vi "Settings Panel.vi"() -> ()   [LabVIEW 2012, in "Scan Driver.lvclass"]
doc: "Main method of the Scan Driver class. Construct a new Scan Driver instance from the given options, or load and deserialize one from an XML file, or modify the last run scan. Configure the instance. Run the scan, and repeat it if more than one scan is requested."
uses:
  Scan Driver.lvclass
  Scanner List.ctl
  Reader List.ctl
  Scan Setup Mode.ctl
  Scan Driver.lvclass/Scan Driver.ctl
  File IO/File IO.lvclass
  Global/File Locations.vi
panel:
  in  "Scanner 2":T1=enum."None"
  in  "Use LCD?":bool
  in  "Based on Last Scan":bool=TRUE
  in  "Path":path
  in  "Scanner":T1
  in  "Reader":T2
  in  "Scan Setup":T3
  out "Update UI":bool
  in  "Continue":bool
  out "error out":errorcluster
  in  "error in (no error)":errorcluster
  in  "exit":bool
  out "dispscan":string caption="Previous Settings"
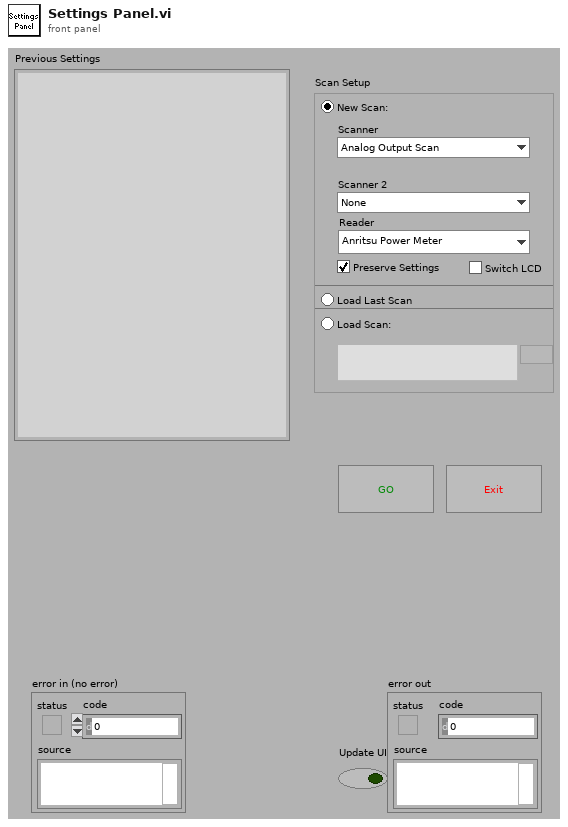
[diagram p1: front panel]
types:
  T1 = typedef "Scan Driver.lvclass/Scanner List.ctl" = enum16{"Analog Output Scan", "Continuous", "Dummy Scan", "Function Gen Scan", "Magnetic Field", "Magna Current Scan", "Magna Voltage Scan", "Microwave Freq Scan", "Pulse Gen Scan", "Pulse Gen Basic Scan", "Translation Stage Dual", "Wavelength", "Wavelength Digikröm", "Wavelength ActiveX", "Translation Stage Coarse", "Translation Stage Fine", "None"}
  T2 = typedef "Scan Driver.lvclass/Reader List.ctl" = enum16{"Anritsu Power Meter", "DAQmx Analog", "Dummy", "Lockin SR830", "Multimeter", "Photon Counter", "Power Meter", "Temperature Control"}
  T3 = typedef "Scan Driver.lvclass/Scan Setup Mode.ctl" = enum32{"New Scan", "Load Last Scan", "Load Scan:"}
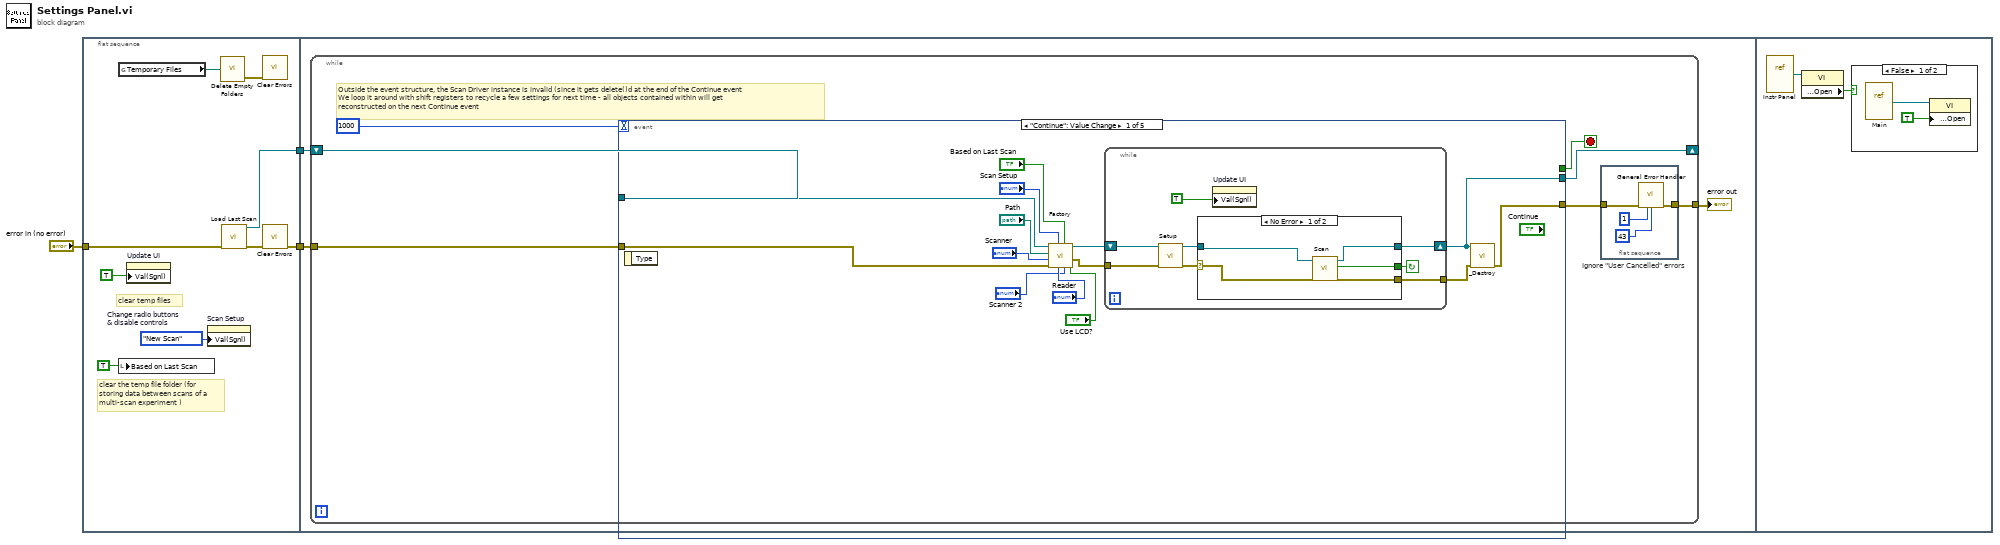
[diagram p0: block diagram]
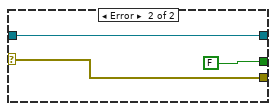
[diagram p2: hidden frame]
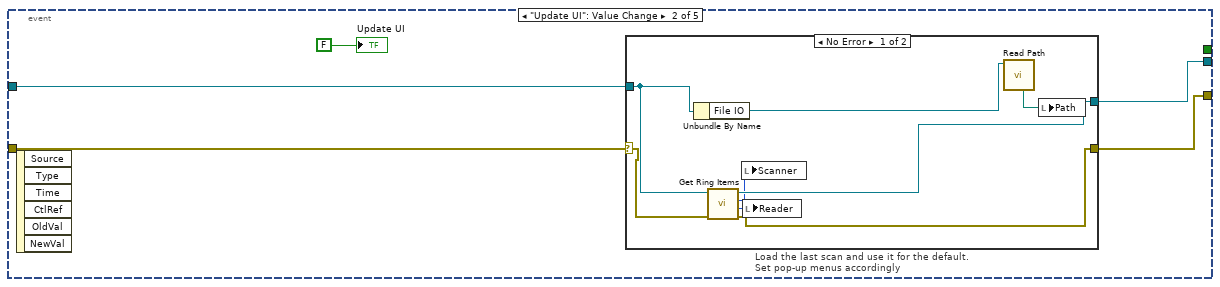
[diagram p3: hidden frame]
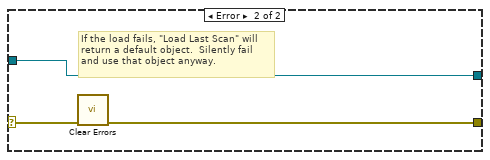
[diagram p4: hidden frame]
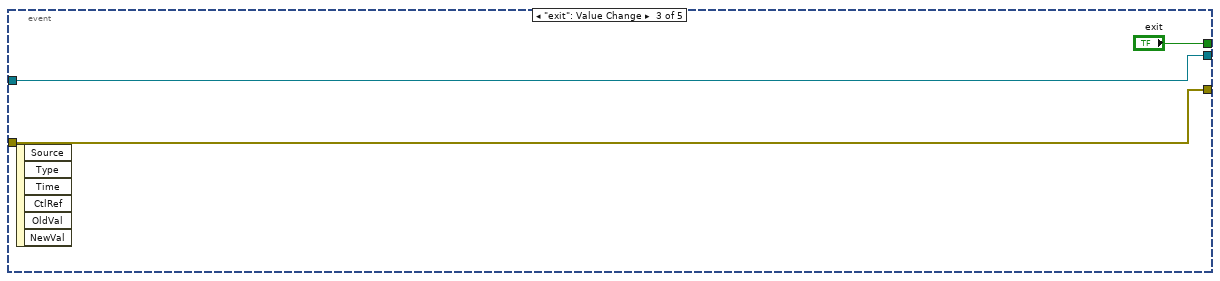
[diagram p5: hidden frame]
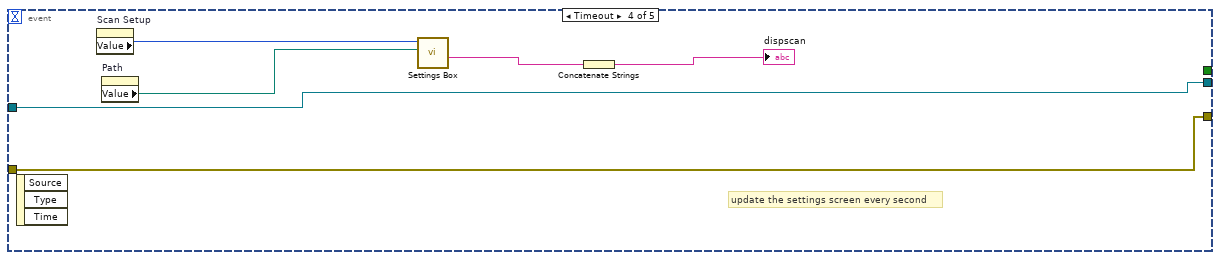
[diagram p6: hidden frame]
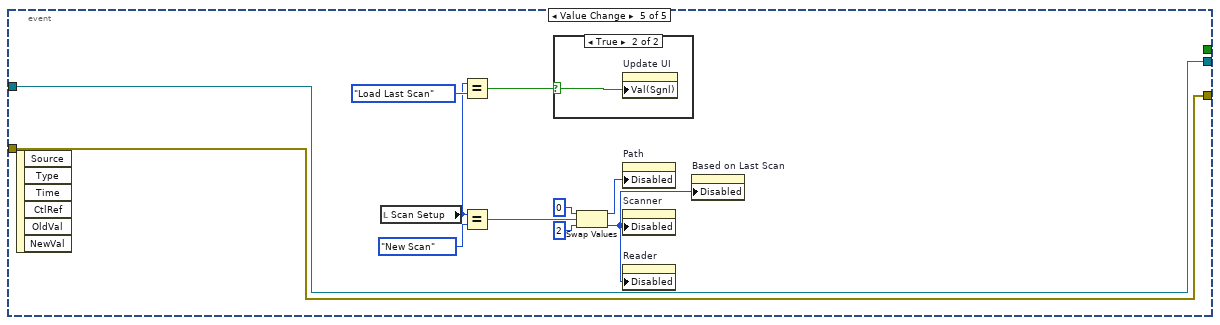
[diagram p7: hidden frame]
diagram:
  n1 = flat-sequence {
    tunnel: "error in (no error)" -> [w10]
    tunnel: [w4] -> w2
    tunnel: [w6] -> w1
    tunnel: w2 -> [w14]
    tunnel: w1 -> [w13]
    frame #0 {
      w8 = Scan_Setup_Mode."New Scan"  # Change radio buttons & disable controls
      # "clear the temp file folder (for storing data between scans of a multi-scan experiment )"
      # "clear temp files"
      n2 = local write "Based on Last Scan"(TRUE ("Based on Last Scan")) -> ()
      n3 = global read "File Locations.vi" "Temporary Files"() -> (w12:path)
      n4 = property on="Update UI" class="Bool (strict)"("Val(Sgnl)"=TRUE ("Value (Signaling)")) -> ()  [unwired: 2 in, 2 out]
      n5 = property on="Scan Setup" class="RadioBtnsControl (strict)"("Val(Sgnl)"=w8) -> ()  [unwired: 2 in, 2 out]
      n6 = call "Delete Empty Folders.vi"("dirpath"=w12) -> ("error out"=w11:errorcluster)  [unwired: 4 out]
      n7 = call "Load Last Scan.vi"("error in"=w10) -> ("error out"=w7:errorcluster, "Last Run Scan"=w6:refnum<class "Scan Driver.lvclass">)  [unwired: 9 out]
      n8 = call <vilib>:"Clear Errors.vi"("error in (no error)"=w11) -> ()  [unwired: 7 out]
      n9 = call <vilib>:"Clear Errors.vi"("error in (no error)"=w7) -> ("error out"=w4:errorcluster)  [unwired: 6 out]
    }
    frame #1 {
      n10 = while {
        shift-right: [w22] -> _
        shift-left: w13 -> [w17]
        tunnel: [w18] -> w15
        tunnel: w14 -> [w16]
        stop <- w21 stop-if-true
        # "Outside the event structure, the Scan Driver instance is invalid (since it gets delete()d at the end of the Continue event\nWe loop it around with shift registers to recycle a few settings for next time - all objects contained within will get\nreconstructed on the next Continue event"
        n11 = event shown="[0] \"Continue\": Value Change" {
          selector: _ -> [_ _ _ _ _]
          dyn-events: _ -> [_ _ _ _ _]
          timeout: 1000 -> [_ _ _ _ _]
          tunnel: [w39 w59 w74 w80 w89] -> w22
          tunnel: [w33 w61 w73 w79 w85] -> w19
          tunnel: w16 -> [w38 w60 w73 w79 w85]
          tunnel: [_ _ "exit" _ _] -> w21
          tunnel: w17 -> [w37 w58 w74 w80 w89]
          event "Continue": Value Change {
            n12 = event-data() -> ()  [unwired: 2 out]
            n13 = call "Factory.vi"("Use LCD?"="Use LCD?", "Scanner 2"="Scanner 2", "Recycle?"="Based on Last Scan", "Reader"="Reader", "Scan Setup Mode"="Scan Setup", "error in"=w38, "Scanner"="Scanner", "Path"="Path", "Recycle old Scan Driver in"=w37) -> ("error out"=w28:errorcluster, "Scan Driver out"=w40:refnum<class "Scan Driver.lvclass">)  [unwired: 1 out]
            n14 = while {
              tunnel: [w43] -> w32
              tunnel: w28 -> [w46]
              shift-right: [w42] -> w39
              shift-left: w40 -> [w47]
              stop <- w45 continue-if-true
              n15 = call-dynamic "Setup.vi"("error in (no error)"=w46, "Scan Driver in"=w47) -> ("error out"=w44:errorcluster, "Scan Driver out"=w48:refnum<class "Scan Driver.lvclass">)  [unwired: 8 out]
              n16 = case shown="No Error" w44 {
                selector: w44 -> [w49 w56]
                tunnel: w48 -> [w50 w55]
                tunnel: [w51 w55] -> w42
                tunnel: [w52 w56] -> w43
                tunnel: [w53 FALSE ("Again?")] -> w45
                frame No Error {
                  n17 = call "Scan.vi"("error in (no error)"=w49, "Scan Driver in"=w50) -> ("error out"=w52:errorcluster, "Again?"=w53:bool, "Scan Driver out"=w51:refnum<class "Scan Driver.lvclass">)  [unwired: 7 out]
                }
                frame Error {
                }
              }
              n18 = property on="Update UI" class="Bool (strict)"("Val(Sgnl)"=TRUE ("Value (Signaling)")) -> ()  [unwired: 2 in, 2 out]
            }
            n19 = call-dynamic "_Destroy.vi"("error in (no error)"=w32, "Scan Driver in"=w39) -> ("error out"=w33:errorcluster)  [unwired: 9 out]
          }
          event "Update UI": Value Change {
            n20 = event-data() -> ()  [unwired: 7 out]
            n21 = case "Load the last scan and use it for the default.  Set pop-up menus accordingly" shown="No Error" w60 {
              selector: w60 -> [w66 w72]
              tunnel: [w67 w70] -> w59
              tunnel: [w65 w71] -> w61
              tunnel: w58 -> [w64 w70]
              frame No Error {
                n22 = Unbundle By Name(w64) -> ("File IO"=w69:refnum<class "File IO.lvclass">)
                n23 = call "Get Ring Items.vi"("error in (no error)"=w66, "Scan Driver in"=w64) -> ("error out"=w65:errorcluster, "Reader"=w62:T2, "Scanner"=w63:T1, "Scan Driver out"=w67:refnum<class "Scan Driver.lvclass">)  [unwired: 6 out]
                n24 = local write "Scanner"(w63) -> ()
                n25 = local write "Reader"(w62) -> ()
                n26 = call-dynamic "Read Path.vi"("File IO.lvclass in"=w69) -> ("Settings Path"=w68:path)  [unwired: 1 in, 9 out]
                n27 = local write "Path"(w68) -> ()
              }
              frame Error {
                # "If the load fails, \"Load Last Scan\" will\nreturn a default object.  Silently fail\nand use that object anyway."
                n28 = call <vilib>:"Clear Errors.vi"("error in (no error)"=w72) -> ("error out"=w71:errorcluster)  [unwired: 6 out]
              }
            }
            "Update UI" <- FALSE ("Update UI")
          }
          event "exit": Value Change {
            n29 = event-data() -> ()  [unwired: 7 out]
          }
          event Timeout {
            # "update the settings screen every second"
            n30 = event-data() -> ()  [unwired: 4 out]
            n31 = property on="Scan Setup" class="RadioBtnsControl (strict)"() -> ("Value"=w77:T3)  [unwired: 2 in, 2 out]
            n32 = property on="Path" class="Path"() -> ("Value"=w76:path)  [unwired: 2 in, 2 out]
            n33 = call "Settings Box.vi"("Path"=w76, "Scan Setup"=w77) -> ("statusbox"=w81:string)  [unwired: 2 in, 7 out]
            n34 = Concatenate Strings(w81) -> (→"dispscan":string)
          }
          event Value Change {
            n35 = event-data() -> ()  [unwired: 7 out]
            n36 = local read "Scan Setup"() -> (w83:T3)
            n37 = Equal?(x=w83, y=Scan_Setup_Mode."Load Last Scan") -> (x = y?=w82:bool)
            n38 = Equal?(x=w83, y=Scan_Setup_Mode."New Scan") -> (x = y?=w88:bool)
            n39 = case shown="True" w82 {
              selector: w82 -> [_ w93]
              frame False {
              }
              frame True {
                n40 = property on="Update UI" class="Bool (strict)"("Val(Sgnl)"=w93) -> ()  [unwired: 2 in, 2 out]
              }
            }
            n41 = Swap Values(12:0 ("x"), 13:w88, 14:2 ("y")) -> (1:w92:i32, 3:w87:i32)
            n42 = property on="Path" class="Path"("Disabled"=w92) -> ()  [unwired: 2 in, 2 out]
            n43 = property on="Scanner" class="Enum (strict)"("Disabled"=w87) -> ()  [unwired: 2 in, 2 out]
            n44 = property on="Reader" class="Enum (strict)"("Disabled"=w87) -> ()  [unwired: 2 in, 2 out]
            n45 = property on="Based on Last Scan" class="Bool (strict)"("Disabled"=w87) -> ()  [unwired: 2 in, 2 out]
          }
        }
        n46 = flat-sequence "Ignore \"User Cancelled\" errors" {
          tunnel: w19 -> [w24]
          tunnel: [w23] -> w18
          frame #0 {
            n47 = call <vilib>:"General Error Handler.vi"("error in (no error)"=w24, "[exception action] (none:0)"=1, "[exception code]"=43) -> ("error out"=w23:errorcluster)  [unwired: 1 in, 11 out]
          }
        }
      }
      "error out" <- w15
    }
    frame #2 {
      n48 = vi-ref "Instr Panel.vi"() -> (w94:refnum<vi>)
      n49 = property class="VI"(reference=w94) -> ("Front Panel Window:Open"=w95:bool)  [unwired: 1 in, 2 out]
      n50 = case shown="False" w95 {
        frame False {
          n51 = vi-ref "Main.vi"() -> (w96:refnum<vi>)
          n52 = property class="VI"(reference=w96, "Front Panel Window:Open"=TRUE) -> ()  [unwired: 1 in, 2 out]
        }
        frame True {
        }
      }
    }
  }
